vi "ContourPlotIntoHistogram V2.5.vi"() -> ()   [LabVIEW 2018]
uses:
  <vilib>/Utility/file.llb/Read Delimited Spreadsheet (DBL).vi
  <vilib>/Utility/file.llb/Write Delimited Spreadsheet (DBL).vi
  <vilib>/Utility/file.llb/Write Delimited Spreadsheet (I64).vi
  <vilib>/Analysis/NI_AALPro.lvlib
panel:
  in  "Specify file name":string
  out "max value":dbl=3.725098
  out "min value":dbl=0.02905273
  out "Progress %":dbl=90.9090909090909
  in  "intervals":i32=4000
  in  "book number":i32=367
  in  "file path (dialog if empty)":path=path "C:/Users/gyue/Box Sync/Guang Yue/data/Contour plot"
  # "Default: Empty"
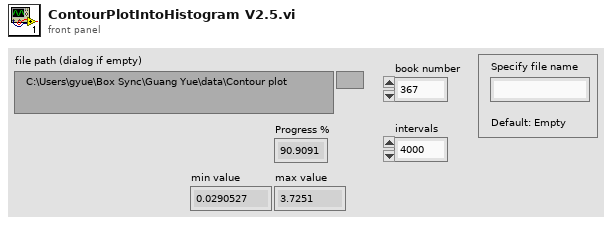
[diagram p1: front panel]
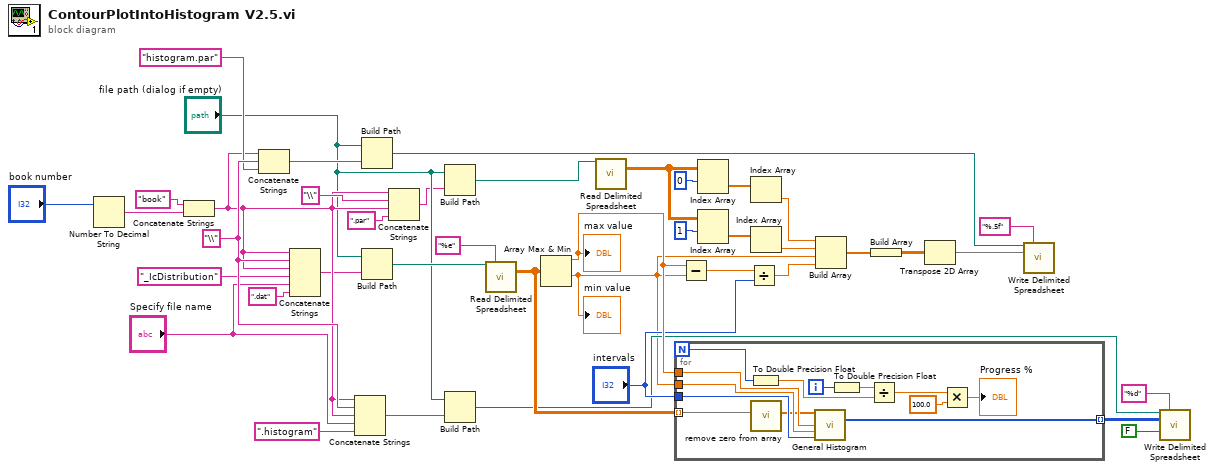
[diagram p0: block diagram]
diagram:
  w28 = "\\" ("string")
  n1 = Number To Decimal String(number="book number") -> (decimal integer string=w41:string)  [unwired: 1 in]
  n2 = Concatenate Strings("book" ("string"), w41) -> (w13:string)
  n3 = Concatenate Strings(w13, w28, "histogram.par" ("string")) -> (w29:string)
  n4 = Concatenate Strings(w13, w28, w13, "_IcDistribution" ("string"), "Specify file name", ".dat" ("string")) -> (w5:string)
  n5 = Concatenate Strings(w13, w28, w13, "Specify file name", ".histogram" ("string")) -> (w4:string)
  n6 = Build Path(base path="file path (dialog if empty)", name or relative path=w29) -> (appended path=w23:path)
  n7 = Build Path(base path="file path (dialog if empty)", name or relative path=w5) -> (appended path=w42:path)
  n8 = Concatenate Strings(w13, "\\" ("string"), w13, ".par" ("string")) -> (w11:string)
  n9 = Build Path(base path="file path (dialog if empty)", name or relative path=w11) -> (appended path=w21:path)
  n10 = Build Path(base path="file path (dialog if empty)", name or relative path=w4) -> (appended path=w31:path)
  n11 = call-poly <vilib>:"Read Delimited Spreadsheet.vi"("file path (dialog if empty)"=w42, "format (%.3f)"="%e") -> ("all rows"=w37:dbl[][])  [unwired: 8 in, 5 out]
  n12 = Array Max & Min(array=w37) -> (max value=w35:dbl, min value=w8:dbl)  [unwired: 2 out]
  "min value" <- w8
  "max value" <- w35
  n13 = call-poly <vilib>:"Read Delimited Spreadsheet.vi"("file path (dialog if empty)"=w21) -> ("all rows"=w14:dbl[][])  [unwired: 9 in, 5 out]
  n14 = for {
    N -> [w50]
    tunnel: w37 -> [w44] mode=indexing
    tunnel: w8 -> [w55]
    tunnel: w35 -> [w54]
    tunnel: "intervals" -> [w53]
    tunnel: [w52] -> w33 mode=indexing
    i -> [w51]
    n15 = To Double Precision Float(number=w50) -> (double precision float=w45:dbl)
    n16 = call "remove zero from array.vi"("in"=w44) -> ("out"=w43:dbl[])  [unwired: 10 in]
    n17 = call <vilib>:"General Histogram.vi"("X"=w43, "max"=w54, "min"=w55, "# bins"=w53) -> ("Histogram"=w52:i32[])  [unwired: 7 in, 4 out]
    n18 = To Double Precision Float(number=w51) -> (double precision float=w46:dbl)
    n19 = Divide(x=w46, y=w45) -> (x/y=w49:dbl)
    n20 = Multiply(x=w49, y=100.0) -> (x*y=→"Progress %":dbl)
  }
  n21 = Subtract(x=w35, y=w8) -> (x-y=w36:dbl)
  n22 = Index Array(array=w14, index (row)=0) -> (element=w18:dbl[])  [unwired: 1 in]
  n23 = Index Array(array=w14, index (row)=1) -> (element=w17:dbl[])  [unwired: 1 in]
  n24 = Divide(x=w36, y="intervals") -> (x/y=w7:dbl)
  n25 = Index Array(array=w18) -> (element=w10:dbl)  [unwired: 1 in]
  n26 = Index Array(array=w17) -> (element=w9:dbl)  [unwired: 1 in]
  n27 = Build Array(w10, w9, w8, w7) -> (w26:dbl[])
  n28 = Build Array(w26) -> (w25:dbl[][])
  n29 = Transpose 2D Array(2D array=w25) -> (transposed array=w24:dbl[][])
  n30 = call-poly <vilib>:"Write Delimited Spreadsheet.vi"("file path (dialog if empty)"=w23, "format (%.3f)"="%.5f", "2D data"=w24) -> ()  [unwired: 11 in, 2 out]
  n31 = call-poly <vilib>:"Write Delimited Spreadsheet.vi"("file path (dialog if empty)"=w31, "format (%d)"="%d", "2D data"=w33, "append to file? (new file:F)"=FALSE) -> ()  [unwired: 10 in, 2 out]
